vi "Aquire Continous Counter Value.vi"() -> ()   [LabVIEW 2020]
uses:
  <instrlib>/BDAQ-6104/Private/Edge Triger Type.ctl
  <instrlib>/BDAQ-6104/Public/Configure/Configure Edge Counter.vi
  <instrlib>/BDAQ-6104/Public/Data/Start Counter.vi
  <instrlib>/BDAQ-6104/Public/Data/Stop Counter.vi
  <instrlib>/BDAQ-6104/BDAQ-6104.lvlib
panel:
  in  "Mode":T1=enum."RISING"
  in  "Reset Count":bool
  in  "VISA resource name":refnum<visa-resource-name>
  out "Count":i32
  in  "stop":bool
  # "Continously queries and displays the counter value.\nThe \"Reset Count\" button will restart the count from 0.\nA counter source must be supplied on port DIO1."
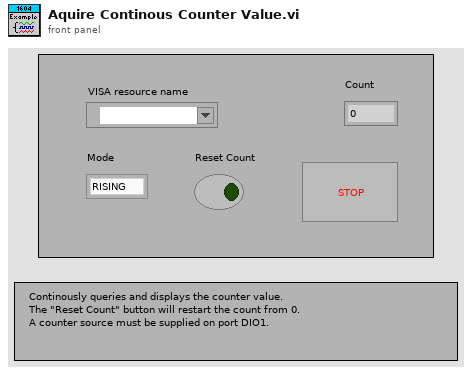
[diagram p1: front panel]
types:
  T1 = typedef "BDAQ-6104.lvlib/Edge Triger Type.ctl" = enum16{"CHANGE", "FALLING", "RISING"}
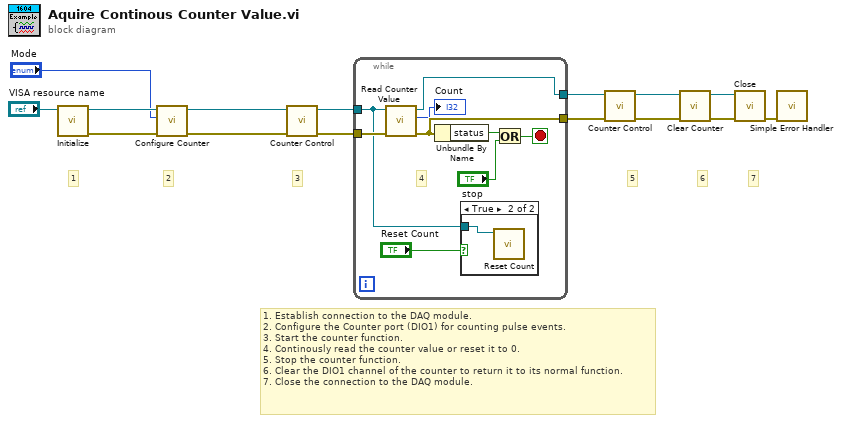
[diagram p0: block diagram]
diagram:
  # "1. Establish connection to the DAQ module.\n2. Configure the Counter port (DIO1) for counting pulse events.\n3. Start the counter function.\n4. Continously read the counter value or reset it to 0.\n5. Stop the counter function.\n6. Clear the DIO1 channel of the counter to return it to its normal function.\n7. Close the connection to the DAQ module."
  # "7"
  # "6"
  # "5"
  # "4"
  # "3"
  # "2"
  # "1"
  n1 = call <instrlib>:"Initialize.vi"("VISA resource name"="VISA resource name") -> ("error out"=w14:errorcluster, "VISA resource name out"=w15:refnum<visa-resource-name>)  [unwired: 9 in]
  n2 = call-poly <instrlib>:"Configure Counter.vi"("error in"=w14, "Mode"="Mode", "VISA resource name"=w15) -> ("error out"=w6:errorcluster, "VISA resource name out"=w9:refnum<visa-resource-name>)  [unwired: 7 in]
  n3 = call-poly <instrlib>:"Counter Control.vi"("error in (no error)"=w6, "VISA resource name"=w9) -> ("error out"=w7:errorcluster, "VISA resource name out"=w8:refnum<visa-resource-name>)  [unwired: 8 in]
  n4 = while {
    tunnel: w8 -> [w17]
    tunnel: w7 -> [w24]
    tunnel: [w23] -> w10
    tunnel: [w21] -> w11
    stop <- w20 stop-if-true
    n5 = call <instrlib>:"Read Counter Value.vi"("error in (no error)"=w24, "VISA resource name"=w17) -> ("error out"=w21:errorcluster, "Count"=→"Count":i32, "VISA resource name out"=w23:refnum<visa-resource-name>)  [unwired: 7 in]
    n6 = Unbundle By Name(w21) -> ("status"=w18:bool)
    n7 = case shown="True" "Reset Count" {
      tunnel: w17 -> [_ w25]
      frame False {
      }
      frame True {
        n8 = call <instrlib>:"Reset Count.vi"("VISA resource name"=w25) -> ()  [unwired: 9 in, 2 out]
      }
    }
    n9 = Or(x=w18, y="stop") -> (x .or. y?=w20:bool)
  }
  n10 = call-poly <instrlib>:"Counter Control.vi"("error in (no error)"=w11, "VISA resource name"=w10) -> ("error out"=w1:errorcluster, "VISA resource name out"=w4:refnum<visa-resource-name>)  [unwired: 8 in]
  n11 = call <instrlib>:"Clear Counter.vi"("error in (no error)"=w1, "VISA resource name"=w4) -> ("error out"=w3:errorcluster, "VISA resource name out"=w2:refnum<visa-resource-name>)  [unwired: 8 in]
  n12 = call <instrlib>:"Close.vi"("error in (no error)"=w3, "VISA resource name"=w2) -> ("error out"=w13:errorcluster)  [unwired: 9 in]
  n13 = call <vilib>:"Simple Error Handler.vi"("error in (no error)"=w13) -> ()  [unwired: 4 in, 5 out]
